vi "clearpath_read_bytestream.vi"(6 "Input Message Buffer":u8[][](array[numeric]) format="%x", 7 "Input Buffer":string="AA01FE43", 8 "Input Read Idx":i32, 9 "Input Write Idx":i32, 10 "Input Num. Char Rem":i32, 11 "Input Char Idx":i32) -> (0 "Output Read Index":u8, 1 "Output Write Index":u8, 2 "Output Num. Char Rem":u8, 3 "Output Char Idx":u8, 4 "Output Message Buffer":u8[][](array[numeric]) format="%x")   [LabVIEW 2009]
uses:
  cwrap_cRIO.dll
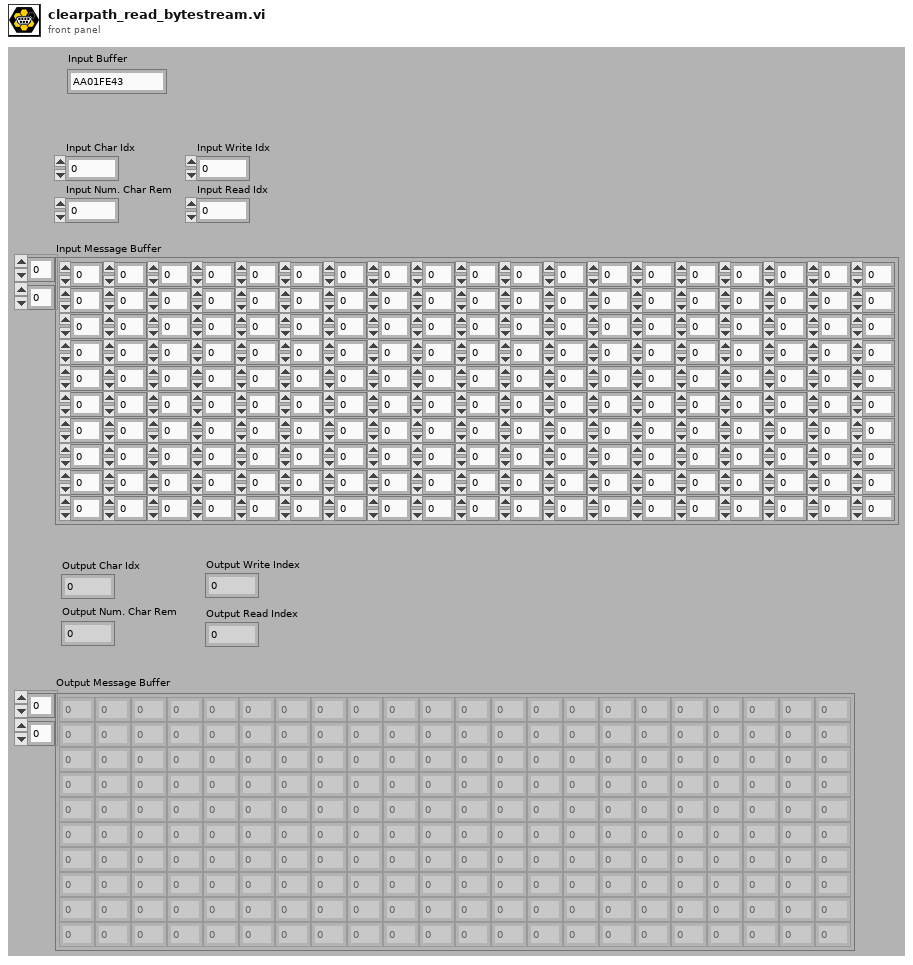
[diagram p1: front panel]
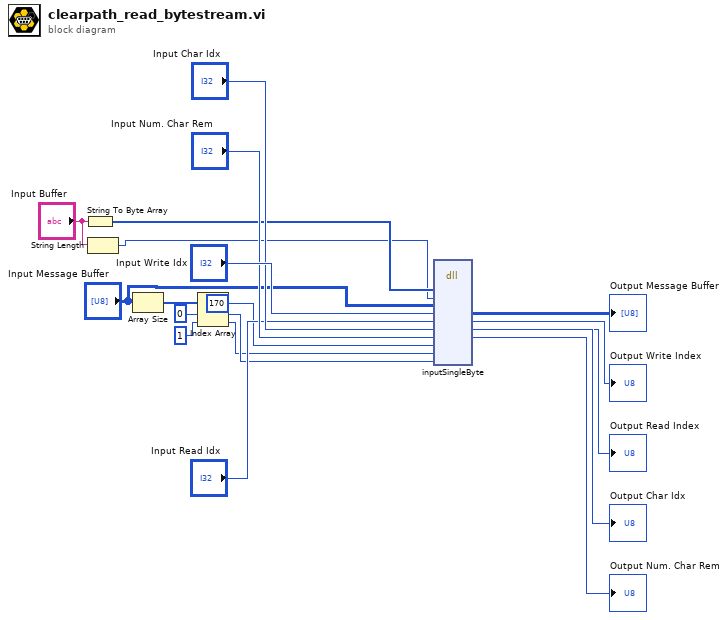
[diagram p0: block diagram]
diagram:
  n1 = String To Byte Array(string="Input Buffer") -> (unsigned byte array=w14:u8[])
  n2 = String Length(string="Input Buffer") -> (length=w6:i32)
  n3 = Array Size(array="Input Message Buffer") -> (size(s)=w11:i32[])
  n4 = Index Array(array=w11, index #1=0 ("index"), index #2=1 ("index")) -> (element #1=w9:i32, element #2=w8:i32)
  n5 = dll-call lib="cwrap_cRIO.*" fn="inputSingleByte"("new_bytes"=w14, "recv_len"=w6, "recv_buffer"="Input Message Buffer", "cur_write_buf"="Input Write Idx", "cur_read_buf"="Input Read Idx", "char_idx"="Input Char Idx", "num_char_left"="Input Num. Char Rem", "SOH"=u8 170, "RECV_LEN"=w8, "NUM_BUF"=w9) -> ("recv_buffer"=→"Output Message Buffer":i8[][], "cur_write_buf"=→"Output Write Index":u8, "cur_read_buf"=→"Output Read Index":u8, "char_idx"=→"Output Char Idx":u8, "num_char_left"=→"Output Num. Char Rem":u8)  [unwired: 9 in, 2 out]
